vi "GNSS Open.vi"(11 "Error In":errorcluster) -> (2 "GNSS Handle":T1, 3 "Error Out":errorcluster)   [LabVIEW 2021]
uses:
  GNSS Handle.ctl
  <vilib>/Instr/_visa.llb/VISA Configure Serial Port (Instr).vi
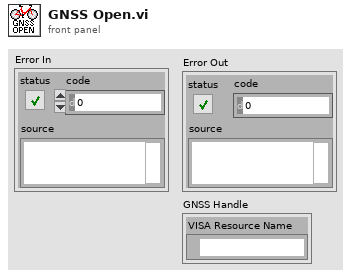
[diagram p1: front panel]
types:
  T1 = typedef "GNSS Handle.ctl" = cluster{"VISA Resource Name":refnum<visa-resource-name>}
  T2 = cluster{"VISA resource name out":refnum<visa-resource-name>}
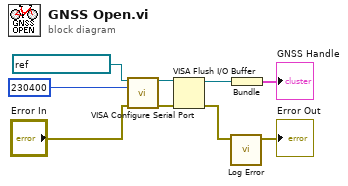
[diagram p0: block diagram]
diagram:
  n1 = call-poly "VISA Configure Serial Port"("VISA resource name"=refnum<visa-resource-name> "ASRL1::INSTR", "baud rate (9600)"=u32 230400, "error in (no error)"="Error In") -> ("VISA resource name out"=w8:refnum<visa-resource-name>, "error out"=w9:errorcluster)  [unwired: 11 in]
  n2 = VISA Flush I/O Buffer(VISA resource name=w8, error in (no error)=w9) -> (VISA resource name out=w4:refnum<visa-resource-name>, error out=w2:errorcluster)  [unwired: 1 in]
  n3 = call "Log Error.vi"("Error In"=w2) -> ("Error Out"=→"Error Out":errorcluster)  [unwired: 10 in]
  n4 = Bundle("VISA resource name out"=w4) -> (→"GNSS Handle":T2)  [unwired: 1 in]
